vi "PulseWidthandFrequency.vi"() -> ()   [LabVIEW 2017]
uses:
  <vilib>/DAQmx/read.llb/DAQmx Read (Counter DBL 1Chan 1Samp).vi
  <vilib>/DAQmx/create/channels.llb/DAQmx Create Channel (CI-Pulse Width).vi
  <vilib>/DAQmx/create/channels.llb/DAQmx Create Channel (CI-Frequency).vi
  <vilib>/DAQmx/miscellaneous.llb/DAQmx Fill In Error Info.vi
  <resource>/objmgr/daqmx.rc
panel:
  out "data":dbl format="%.3p"
  in  "counter":tag="Dev6/ctr0"
  in  "?":enum32{"Pulse Width", "Frequency"}(tab)
  in  "CI.PulseWidth.Term":tag="/Dev6/PFI15"
  in  "CI.Freq.Term":tag="/Dev6/PFI15"
  in  "stop":bool
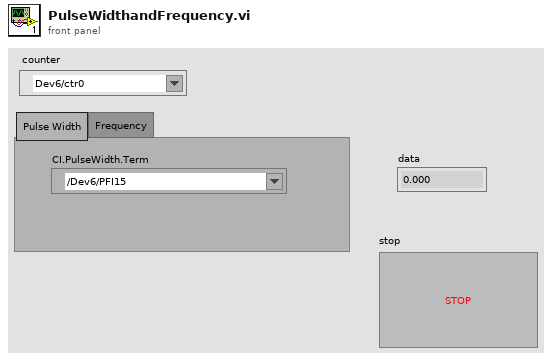
[diagram p1: front panel]
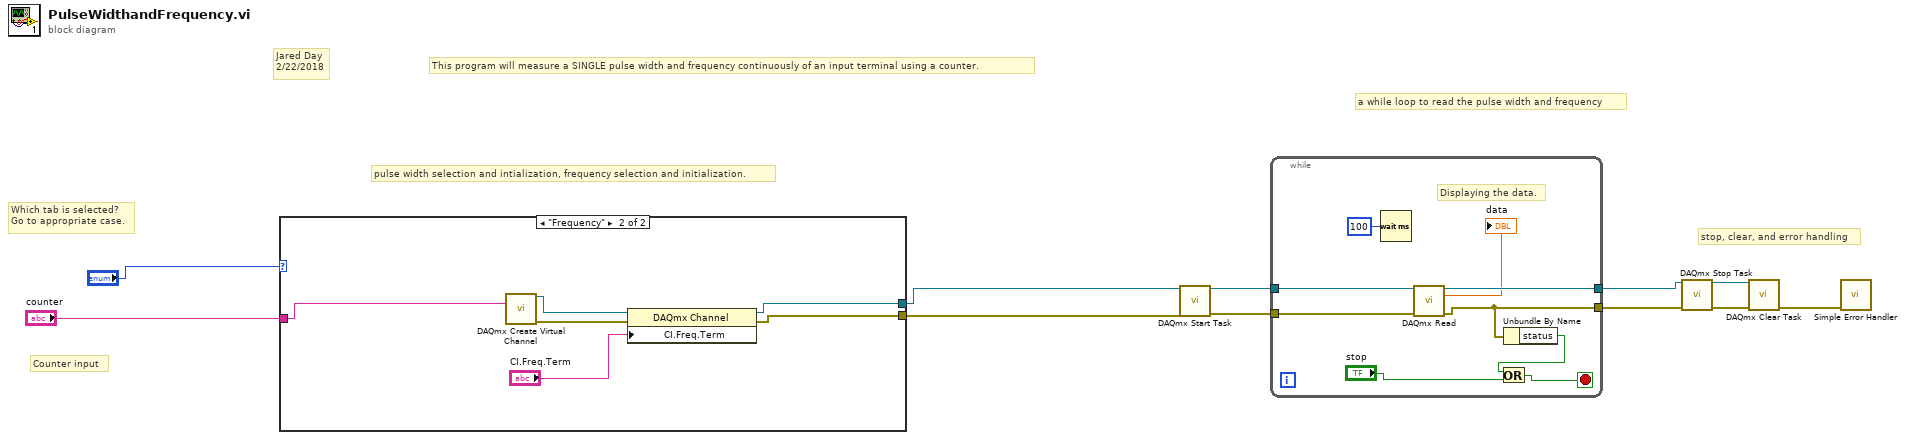
[diagram p0: block diagram]
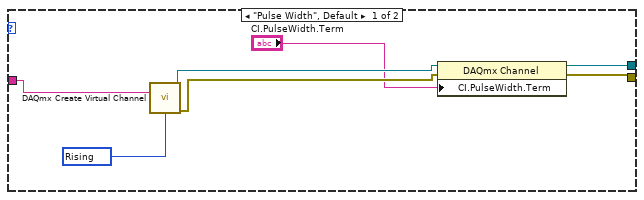
[diagram p2: hidden frame]
diagram:
  # "stop, clear, and error handling"
  # "a while loop to read the pulse width and frequency"
  # "pulse width selection and intialization, frequency selection and initialization."
  # "Counter input"
  # "Which tab is selected?\nGo to appropriate case."
  # "This program will measure a SINGLE pulse width and frequency continuously of an input terminal using a counter."
  # "Jared Day\n2/22/2018"
  n1 = case shown="\"Frequency\"" "?" {
    tunnel: "counter" -> [w15 w24]
    tunnel: [w14 w20] -> w2
    tunnel: [w13 w19] -> w1
    frame "Pulse Width", Default {
      w12 = 10280 items=["Rising"=10280, "Falling"=10171] ("starting edge")
      n2 = call-poly <vilib>:"DAQmx Create Virtual Channel.vi"("counter"=w15, "starting edge"=w12) -> ("task out"=w18:refnum<k21>, "error out"=w17:errorcluster)  [unwired: 12 in]
      n3 = property class="DAQmx Channel"(reference=w18, error in=w17, "CI.PulseWidth.Term"="CI.PulseWidth.Term") -> (reference out=w14:refnum<k21>, error out=w13:errorcluster)
    }
    frame "Frequency" {
      n4 = call-poly <vilib>:"DAQmx Create Virtual Channel.vi"("counter"=w24) -> ("task out"=w23:refnum<k21>, "error out"=w22:errorcluster)  [unwired: 13 in]
      n5 = property class="DAQmx Channel"(reference=w23, error in=w22, "CI.Freq.Term"="CI.Freq.Term") -> (reference out=w20:refnum<k21>, error out=w19:errorcluster)
    }
  }
  n6 = call <vilib>:"DAQmx Start Task.vi"("task/channels in"=w2, "error in"=w1) -> ("task out"=w6:refnum<k21>, "error out"=w5:errorcluster)  [unwired: 12 in]
  n7 = while {
    tunnel: w6 -> [w33]
    tunnel: w5 -> [w32]
    tunnel: [w30] -> w4
    tunnel: [w31] -> w3
    stop <- w29 stop-if-true
    # "Displaying the data."
    n8 = Wait (ms)(milliseconds to wait=u32 100) -> ()  [unwired: 1 out]
    n9 = call-poly <vilib>:"DAQmx Read.vi"("task/channels in"=w33, "error in"=w32) -> ("task out"=w31:refnum<k21>, "data"=→"data":dbl, "error out"=w30:errorcluster)  [unwired: 11 in]
    n10 = Unbundle By Name(w30) -> ("status"=w27:bool)
    n11 = Or(x=w27, y="stop") -> (x .or. y?=w29:bool)
  }
  n12 = call <vilib>:"DAQmx Stop Task.vi"("task/channels in"=w3, "error in"=w4) -> ("task out"=w9:refnum<k21>, "error out"=w8:errorcluster)  [unwired: 12 in]
  n13 = call <vilib>:"DAQmx Clear Task.vi"("task in"=w9, "error in"=w8) -> ("error out"=w7:errorcluster)  [unwired: 13 in]
  n14 = call <vilib>:"Simple Error Handler.vi"("error in (no error)"=w7) -> ()  [unwired: 4 in, 5 out]
